vi "Copy from Public to Server.vi"(7 "Archive File?":bool[](array[boolean]), 8 "error in (no error)":errorcluster, 9 "Running on Server?":bool, 10 "Path of Files relative to EnFlo Data Root":path[](array[path]), 11 "Application in":refnum<vi>) -> (0 "error out":errorcluster)   [LabVIEW 2015]
uses:
  Harvest_Global.vi
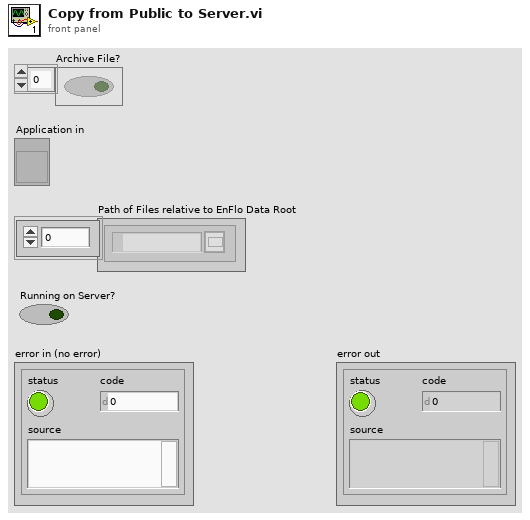
[diagram p1: front panel]
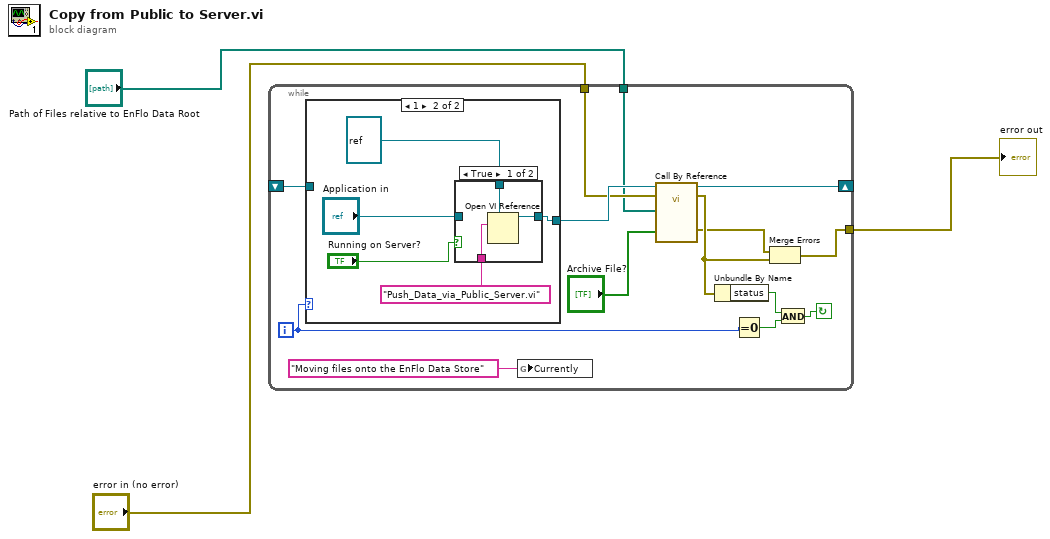
[diagram p0: block diagram]
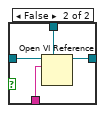
[diagram p3: hidden frame]
diagram:
  n1 = while {
    shift-right: [w15] -> _
    shift-left: _ -> [w17]
    tunnel: [w5] -> w3
    tunnel: "error in (no error)" -> [w9]
    tunnel: "Path of Files relative to EnFlo Data Root" -> [w8]
    i -> [w14]
    stop <- w11 continue-if-true
    n2 = case shown="1" w14 {
      tunnel: w17 -> [w18 _]
      tunnel: [w18 w23] -> w16
      frame 0, Default {
      }
      frame 1 {
        n3 = case shown="True" "Running on Server?" {
          tunnel: [w26 w30] -> w23
          tunnel: "Application in" -> [_ w29]
          tunnel: refnum<vi> refnum ("Push Data Server") -> [w25 w28]
          tunnel: "Push_Data_via_Public_Server.vi" -> [w24 w27]
          frame True {
            n4 = Open VI Reference(type specifier VI Refnum (for type only)=w25, vi path=w24) -> (vi reference=w26:refnum<vi>)  [unwired: 2 in, 3 out]
          }
          frame False {
            n5 = Open VI Reference(type specifier VI Refnum (for type only)=w28, application reference (local)=w29, vi path=w27) -> (vi reference=w30:refnum<vi>)  [unwired: 1 in, 3 out]
          }
        }
      }
    }
    n6 = global write "Harvest_Global.vi" "Currently"("Moving files onto the EnFlo Data Store" ("Currently Running")) -> ()
    n7 = call-by-ref "?"(reference=w16, error in=w9, "Archive File?"="Archive File?", "Path of Files relative to EnFlo Data Root"=w8) -> (reference out=w15:refnum<vi>, error out=w7:errorcluster, "error out"=w6:errorcluster)  [unwired: 2 in]
    n8 = Unbundle By Name(w7) -> ("status"=w12:bool)
    n9 = Equal To 0?(x=w14) -> (x = 0?=w13:bool)
    n10 = Merge Errors(w6, w7) -> (w5:errorcluster)
    n11 = And(x=w12, y=w13) -> (x .and. y?=w11:bool)
  }
  "error out" <- w3
